vi "Query Generator Dual Tone Output Level.vi"(8 "error in (no error)":errorcluster, 9 "Source (1)":i32=1 format="%.0g", 10 "Instance (1)":i32=1 format="%.0g", 11 "VISA resource name":refnum<visa-resource-name>) -> (0 "error out":errorcluster, 2 "Output Level":dbl format="%^.3e", 3 "VISA resource name out":refnum<visa-resource-name>)   [LabVIEW 2015, in "Rohde&Schwarz CMXP GPRF.lvlib"]
doc: "Queries the output level of the source signal <source>. The output level is a VI of the generator output level and the ratio.\n\nAttribute:\nRSCMXPGPRF_ATTR_DUAL_TONE_LEVEL\n\nRemote-control command:\nSOURce:GPRF:GEN<i>:DTONe:LEVel<source>?"
uses:
  <instrlib>/Rohde&Schwarz CMXP GPRF/Rohde&Schwarz CMXP GPRF.lvlib
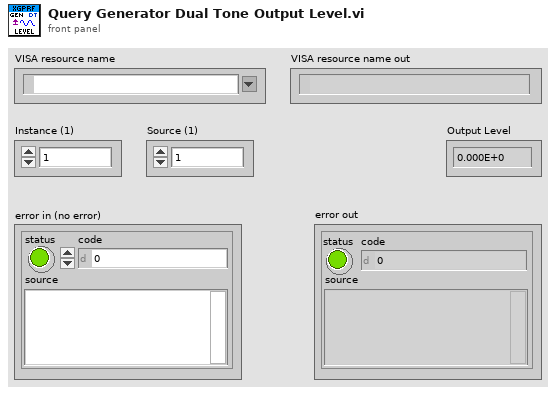
[diagram p1: front panel]
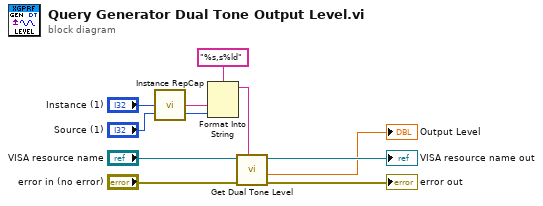
[diagram p0: block diagram]
diagram:
  n1 = call <instrlib>:"Instance RepCap.vi"("instance  in"="Instance (1)") -> ("instance out"=w8:string)
  n2 = Format Into String(format string="%s,s%ld", w8, "Source (1)") -> (resulting string=w9:string)  [unwired: 2 in, 1 out]
  n3 = call "Get Dual Tone Level"("Repeated Capabilities"=w9, "error in (no error)"="error in (no error)", "instrument handle"="VISA resource name") -> ("error out"=→"error out":errorcluster, "Dual Tone Level"=→"Output Level":dbl, "instrument handle out"=→"VISA resource name out":refnum<visa-resource-name>)  [unwired: 6 in]
